vi "demo.vi"() -> ()   [LabVIEW 2013]
uses:
  Gum Machine_class/Gum Machine.lvclass
  <vilib>/addons/_AddQ/G#Object/G#Object.lvclass
panel:
  in  "设定货物数量":u32
  out "库存货物数量":u32
  out "Output":string
  in  "停止":bool
  in  "转动曲柄":bool
  in  "退币":bool
  in  "投币":bool
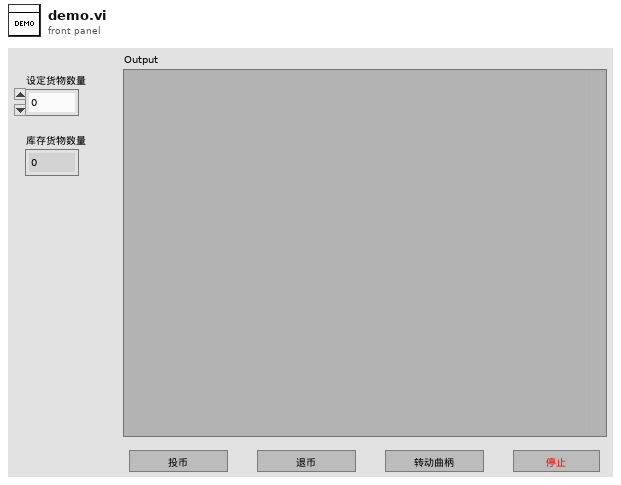
[diagram p1: front panel]
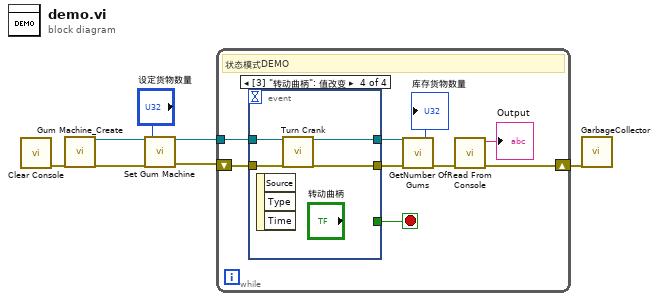
[diagram p0: block diagram]
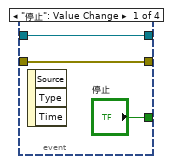
[diagram p2: hidden frame]
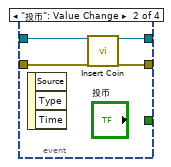
[diagram p3: hidden frame]
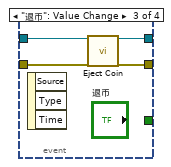
[diagram p4: hidden frame]
diagram:
  n1 = call "Clear Console.vi"() -> ("error out"=w5:errorcluster)  [unwired: 11 in]
  n2 = call "Gum Machine_Create.vi"("error in (no error)"=w5) -> ("reference out"=w7:refnum<class "Gum Machine.lvclass">, "error out"=w6:errorcluster)  [unwired: 17 in]
  n3 = call "Set Gum Machine.vi"("reference in"=w7, "error in (no error)"=w6, "Number Of Gums"="设定货物数量") -> ("reference out"=w2:refnum<class "Gum Machine.lvclass">, "error out"=w1:errorcluster)  [unwired: 15 in]
  n4 = while {
    tunnel: w2 -> [w15]
    shift-right: [w12] -> w4
    shift-left: w1 -> [w14]
    stop <- w16 stop-if-true
    # "状态模式DEMO"
    n5 = event shown="[3] \"转动曲柄\": 值改变" {
      selector: _ -> [_ _ _ _]
      dyn-events: _ -> [_ _ _ _]
      timeout: _ -> [_ _ _ _]
      tunnel: ["停止" _ _ _] -> w16
      tunnel: w15 -> [w17 w22 w26 w29]
      tunnel: w14 -> [w18 w23 w27 w31]
      tunnel: [w18 w21 w25 w30] -> w11
      tunnel: [w17 w20 w24 w28] -> w10
      event "停止": Value Change {
        n6 = event-data() -> ()  [unwired: 1 in, 3 out]
      }
      event "投币": Value Change {
        n7 = event-data() -> ()  [unwired: 1 in, 3 out]
        n8 = call-dynamic "Insert Coin.vi"("reference in"=w22, "error in (no error)"=w23) -> ("reference out"=w20:refnum<class "Gum Machine.lvclass">, "error out"=w21:errorcluster)  [unwired: 16 in]
      }
      event "退币": Value Change {
        n9 = event-data() -> ()  [unwired: 1 in, 3 out]
        n10 = call-dynamic "Eject Coin.vi"("reference in"=w26, "error in (no error)"=w27) -> ("reference out"=w24:refnum<class "Gum Machine.lvclass">, "error out"=w25:errorcluster)  [unwired: 16 in]
      }
      event "转动曲柄": Value Change {
        n11 = event-data() -> ()  [unwired: 1 in, 3 out]
        n12 = call-dynamic "Turn Crank.vi"("reference in"=w29, "error in (no error)"=w31) -> ("reference out"=w28:refnum<class "Gum Machine.lvclass">, "error out"=w30:errorcluster)  [unwired: 16 in]
      }
    }
    n13 = call-dynamic "GetNumber Of Gums.vi"("error in (no error)"=w11, "reference in"=w10) -> ("error out"=w8:errorcluster, "Number Of Gums"=→"库存货物数量":u32)  [unwired: 7 in, 1 out]
    n14 = call "Read From Console.vi"("error in (no error)"=w8) -> ("error out"=w12:errorcluster, "Output"=→"Output":string)  [unwired: 9 in]
  }
  n15 = call <vilib>:"GarbageCollector.vi"("error in (no error)"=w4) -> ()  [unwired: 16 in, 3 out]
